vi "V7310.Main.Start.vi"(8 "error in":errorcluster, 10 "Job":T1, 11 "Data in":T3={"Status"={"State"=enum."Init", "LaserStatus"=enum."-", "LaserStatusRaw"="", "Ref"=refnum, "RTC TS"=timestamp(0 s since 1904-01-01), "Conn TS"=timestamp(0 s since 1904-01-01), "Msg"=[], "JobInUse"="", "Jobs"=[], "Vars"=[]}, "Sets"={"Address"="192.168.2.1", "Timeout_ms"=5000, "ReconnectPeriod_s"=0, "JobInUse"="", "CoordinatesOffset"={"X"=0.0, "Y"=0.0}}}) -> (0 "error out":errorcluster, 3 "Data out":T3={"Status"={"State"=enum."Init", "LaserStatus"=enum."-", "LaserStatusRaw"="", "Ref"=refnum, "RTC TS"=timestamp(0 s since 1904-01-01), "Conn TS"=timestamp(0 s since 1904-01-01), "Msg"=[], "JobInUse"="", "Jobs"=[], "Vars"=[]}, "Sets"={"Address"="192.168.2.1", "Timeout_ms"=5000, "ReconnectPeriod_s"=0, "JobInUse"="", "CoordinatesOffset"={"X"=0.0, "Y"=0.0}}})   [LabVIEW 2015]
uses:
  V7310.Data.ctl
  V7310.Data.Status.ctl
  V7310.Data.Status.State.ctl
  LowLevel/V7310.LaserStatus.ctl
  LowLevel/V7310.Message.Data.ctl
  LowLevel/V7310.Job.Variable.ctl
  V7310.Data.Sets.ctl
  LowLevel/V7310.Job.Data.ctl
  LowLevel/V7310.Job.Sets.ctl
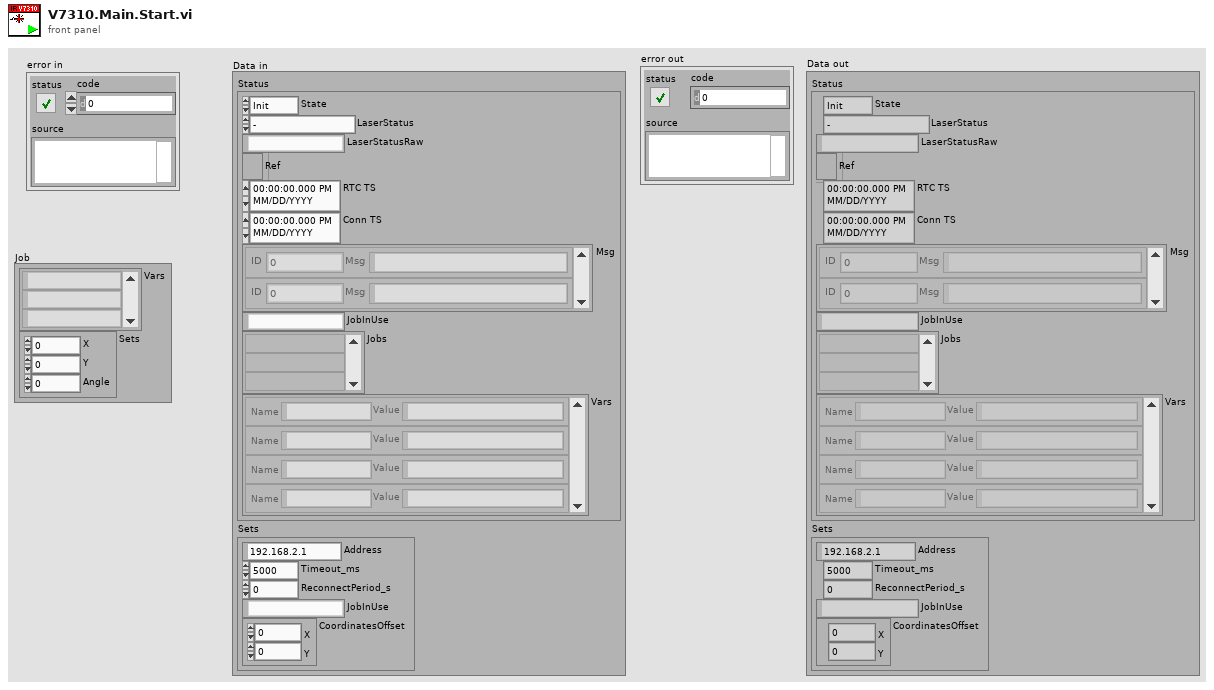
[diagram p1: front panel]
types:
  T1 = typedef "V7310.Job.Data.ctl" = cluster{"Vars":string[], "Sets":T2}
  T2 = typedef "V7310.Job.Sets.ctl" = cluster{"X":dbl, "Y":dbl, "Angle":dbl}
  T3 = typedef "V7310.Data.ctl" = cluster{"Status":T4, "Sets":T9}
  T4 = typedef "V7310.Data.Status.ctl" = cluster{"State":T5, "LaserStatus":T6, "LaserStatusRaw":string, "Ref":refnum<k5>, "RTC TS":timestamp, "Conn TS":timestamp, "Msg":T7[], "JobInUse":string, "Jobs":string[], "Vars":T8[]}
  T5 = typedef "V7310.Data.Status.State.ctl" = enum16{"First", "Init", "Msg", "Error", "Abort", "Idle", "Run"}
  T6 = typedef "V7310.LaserStatus.ctl" = enum16{"-", "FatalError", "Initialize", "KeySwitchOpen", "TimeoutInterlock", "InterlockOpen", "StartUp", "ShutterlockOpen", "Standby", "Ready", "PrepareForMarking", "WaitForTrigger", "Marking"}
  T7 = typedef "V7310.Message.Data.ctl" = cluster{"ID":i32, "Msg":string}
  T8 = typedef "V7310.Job.Variable.ctl" = cluster{"Name":string, "Value":string}
  T9 = typedef "V7310.Data.Sets.ctl" = cluster{"Address":string, "Timeout_ms":i32, "ReconnectPeriod_s":i32, "JobInUse":string, "CoordinatesOffset":cluster{"X":dbl, "Y":dbl}}
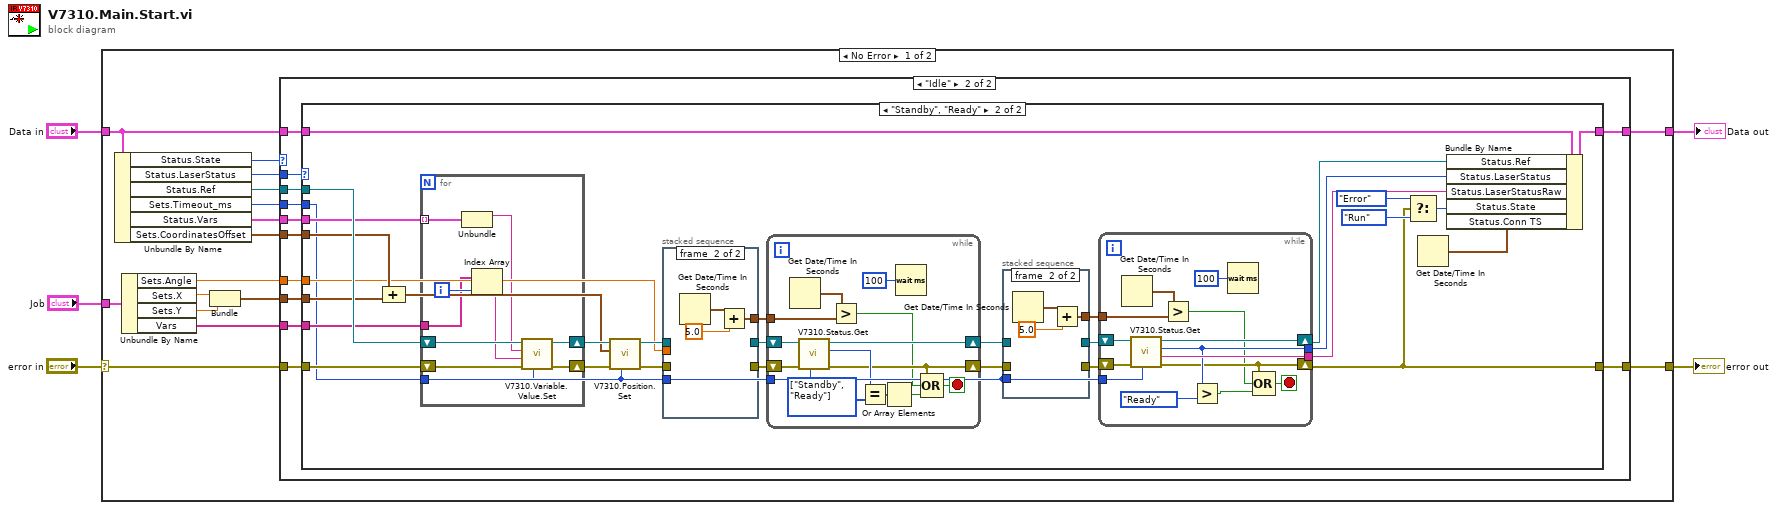
[diagram p0: block diagram]
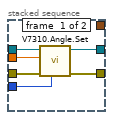
[diagram p4: hidden frame]
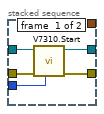
[diagram p5: hidden frame]
diagram:
  n1 = case shown="No Error" "error in" {
    selector: "error in" -> [w18 w125]
    tunnel: [w19 w125] -> w4
    tunnel: "Data in" -> [w20 w124]
    tunnel: [w21 w124] -> w2
    tunnel: "Job" -> [w13 _]
    frame No Error {
      n2 = Unbundle By Name(w20) -> ("Status.State"=w15:T5, "Status.LaserStatus"=w14:T6, "Status.Ref"=w16:refnum<k5>, "Sets.Timeout_ms"=w17:i32, "Status.Vars"=w10:T8[], "Sets.CoordinatesOffset"=w6:cluster{"X":dbl, "Y":dbl})
      n3 = Unbundle By Name(w13) -> ("Sets.Angle"=w12:dbl, "Sets.X"=w9:dbl, "Sets.Y"=w8:dbl, "Vars"=w11:string[])
      n4 = Bundle("X"=w9, "Y"=w8) -> (w7:cluster{"X":dbl, "Y":dbl})  [unwired: 1 in]
      n5 = case shown="\"Idle\"" w15 {
        tunnel: [w23 w35] -> w21
        tunnel: w20 -> [w23 w34]
        tunnel: [w22 w33] -> w19
        tunnel: w18 -> [w22 w32]
        tunnel: w17 -> [_ w30]
        tunnel: w16 -> [_ w31]
        tunnel: w14 -> [_ w29]
        tunnel: w12 -> [_ w28]
        tunnel: w7 -> [_ w27]
        tunnel: w11 -> [_ w26]
        tunnel: w10 -> [_ w25]
        tunnel: w6 -> [_ w24]
        frame Default {
        }
        frame "Idle" {
          n6 = case shown="\"Standby\", \"Ready\"" w29 {
            tunnel: [w37 w68] -> w35
            tunnel: w34 -> [w37 w67]
            tunnel: [w36 w57] -> w33
            tunnel: w32 -> [w36 w62]
            tunnel: w31 -> [_ w61]
            tunnel: w30 -> [_ w39]
            tunnel: w28 -> [_ w40]
            tunnel: w27 -> [_ w60]
            tunnel: w26 -> [_ w59]
            tunnel: w25 -> [_ w49]
            tunnel: w24 -> [_ w47]
            frame Default {
            }
            frame "Standby", "Ready" {
              n7 = Compound Arithmetic op=ADD(w47, w60) -> (w48:cluster{"X":dbl, "Y":dbl})
              n8 = for {
                tunnel: w39 -> [w99]
                shift-right: [w100] -> w51
                shift-left: w61 -> [w101]
                shift-right: [w98] -> w50
                shift-left: w62 -> [w97]
                tunnel: w59 -> [w92]
                tunnel: w49 -> [w96] mode=indexing
                i -> [w93]
                n9 = Unbundle(w96) -> ("Name"=w94:string)  [unwired: 1 out]
                n10 = Index Array(array=w92, index=w93) -> (element=w95:string)
                n11 = call "V7310.Variable.Value.Set.vi"("timeout ms (5000)"=w99, "error in"=w97, "Value"=w95, "Variable"=w94, "Connection in"=w101) -> ("error out"=w98:errorcluster, "Connection out"=w100:refnum<k5>)  [unwired: 5 in]
              }
              n12 = call "V7310.Position.Set.vi"("timeout ms (5000)"=w39, "error in"=w50, "Position"=w48, "Connection in"=w51) -> ("error out"=w44:errorcluster, "Connection out"=w41:refnum<k5>)  [unwired: 6 in]
              n13 = stacked-sequence {
                tunnel: w40 -> [w74 _]
                tunnel: w44 -> [w73 _]
                tunnel: w41 -> [w72 _]
                tunnel: w39 -> [w71 _]
                tunnel: [w70 _] -> w42
                tunnel: [w69 _] -> w43
                tunnel: [_ w75] -> w38
                frame #0 {
                  n14 = call "V7310.Angle.Set.vi"("timeout ms (5000)"=w71, "error in"=w73, "Angle"=w74, "Connection in"=w72) -> ("error out"=w69:errorcluster, "Connection out"=w70:refnum<k5>)  [unwired: 6 in]
                }
                frame #1 {
                  n15 = Get Date/Time In Seconds() -> (seconds since 1Jan1904=w76:timestamp)
                  n16 = Add(x=w76, y=5.0) -> (x+y=w75:timestamp)
                }
              }
              n17 = while {
                shift-right: [w85] -> w45
                shift-left: w43 -> [w91]
                shift-right: [w89] -> w46
                shift-left: w42 -> [w90]
                tunnel: w38 -> [w82]
                tunnel: w39 -> [w78]
                stop <- w84 stop-if-true
                w80 = T6[] [enum."Standby", enum."Ready"] items=["-", "FatalError", "Initialize", "KeySwitchOpen", "TimeoutInterlock", "InterlockOpen", "StartUp", "ShutterlockOpen", "Standby", "Ready", "PrepareForMarking", "WaitForTrigger", "Marking"]
                n18 = Get Date/Time In Seconds() -> (seconds since 1Jan1904=w83:timestamp)
                n19 = call "V7310.Status.Get.vi"("timeout ms (5000)"=w78, "error in"=w91, "Connection in"=w90) -> ("error out"=w85:errorcluster, "LaserStatus"=w87:T6, "Connection out"=w89:refnum<k5>)  [unwired: 5 in, 1 out]
                n20 = Greater?(x=w83, y=w82) -> (0:w81:bool)
                n21 = Equal?(x=w87, y=w80) -> (x = y?=w86:bool[])
                n22 = Or Array Elements(Boolean array=w86) -> (logical OR=w79:bool)
                n23 = Wait (ms)(milliseconds to wait=u32 100) -> ()  [unwired: 1 out]
                n24 = Compound Arithmetic op=OR(w85, w81, w79) -> (w84:bool)
              }
              n25 = stacked-sequence {
                tunnel: w45 -> [w106 _]
                tunnel: w46 -> [w105 _]
                tunnel: w39 -> [w104 _]
                tunnel: [w103 _] -> w58
                tunnel: [w102 _] -> w56
                tunnel: [_ w107] -> w52
                frame #0 {
                  n26 = call "V7310.Start.vi"("timeout ms (5000)"=w104, "error in"=w106, "Connection in"=w105) -> ("error out"=w103:errorcluster, "Connection out"=w102:refnum<k5>)  [unwired: 7 in]
                }
                frame #1 {
                  n27 = Get Date/Time In Seconds() -> (seconds since 1Jan1904=w109:timestamp)
                  n28 = Add(x=w109, y=5.0) -> (x+y=w107:timestamp)
                }
              }
              n29 = while {
                tunnel: [w118] -> w54
                tunnel: [w120] -> w53
                shift-right: [w117] -> w57
                shift-left: w58 -> [w123]
                shift-right: [w121] -> w55
                shift-left: w56 -> [w122]
                tunnel: w52 -> [w114]
                tunnel: w39 -> [w112]
                stop <- w116 stop-if-true
                n30 = Get Date/Time In Seconds() -> (seconds since 1Jan1904=w115:timestamp)
                n31 = call "V7310.Status.Get.vi"("timeout ms (5000)"=w112, "error in"=w123, "Connection in"=w122) -> ("error out"=w117:errorcluster, "Laser Status"=w120:string, "LaserStatus"=w118:T6, "Connection out"=w121:refnum<k5>)  [unwired: 5 in]
                n32 = Greater?(x=w115, y=w114) -> (0:w113:bool)
                n33 = Greater?(x=w118, y=V7310.LaserStatus."Ready") -> (0:w110:bool)
                n34 = Wait (ms)(milliseconds to wait=u32 100) -> ()  [unwired: 1 out]
                n35 = Compound Arithmetic op=OR(w117, w113, w110) -> (w116:bool)
              }
              n36 = Select(t=V7310.Data.Status.State."Error" ("Status.State"), s=w57, f=V7310.Data.Status.State."Run" ("Status.State")) -> (s? t:f=w64:T5)
              n37 = Get Date/Time In Seconds() -> (seconds since 1Jan1904=w63:timestamp)
              n38 = Bundle By Name(cluster=w67, "Status.Ref"=w55, "Status.LaserStatus"=w54, "Status.LaserStatusRaw"=w53, "Status.State"=w64, "Status.Conn TS"=w63) -> (w68:T3)
            }
          }
        }
      }
    }
    frame Error {
    }
  }
  "error out" <- w4
  "Data out" <- w2
